vi "FPGANic.Globals.vi"() -> ()   [LabVIEW 2018]
panel:
  out "FPGA VI Reference Out":refnum<k20>
  in  "IPv4 Message Counter":i16
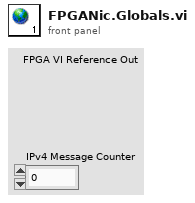
[diagram p1: front panel]
diagram:
